vi "recv.vi"(8 "error in (no error)":errorcluster, 11 "tcp socket fd":i32) -> (0 "error out":errorcluster, 3 "bytes processed":u16)   [LabVIEW 2015]
panel:
  in  "buffer":string
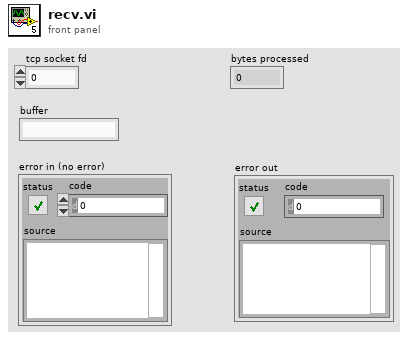
[diagram p1: front panel]
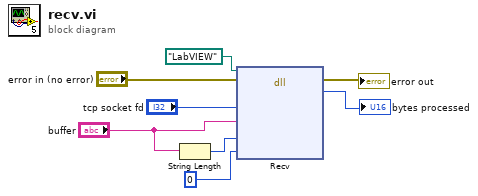
[diagram p0: block diagram]
diagram:
  n1 = String Length(string="buffer") -> (length=w2:i32)
  n2 = dll-call lib="LabVIEW" fn="Recv"(path in=path "LabVIEW", error in="error in (no error)", "sockfd"="tcp socket fd", "buf"="buffer", "len"=w2, "flags"=u16 0) -> (error out=→"error out":errorcluster, "bytesProcessed"=→"bytes processed":i16)  [unwired: 5 in, 1 out]
